vi "stopAllThreads.vi"(0 "HGF_ThreadPool":refnum<class "HGF_ThreadPool.lvclass">, 5 "error in (no error)":errorcluster) -> (14 "dup HGF_ThreadPool":refnum<class "HGF_ThreadPool.lvclass">, 19 "error out":errorcluster)   [LabVIEW 2014, in "HGF_BaseClasses.lvlib" / "HGF_ThreadPool.lvclass"]
doc: "Stop all threads of this ThreadPool."
uses:
  HGF_ThreadPool.lvclass
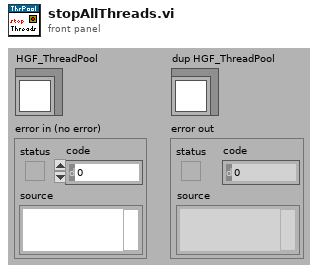
[diagram p1: front panel]
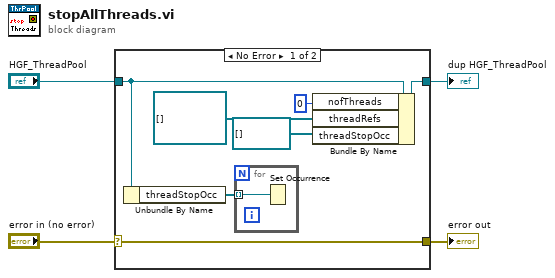
[diagram p0: block diagram]
diagram:
  n1 = case shown="No Error" "error in (no error)" {
    selector: "error in (no error)" -> [w11 w14]
    tunnel: [w11 w14] -> w3
    tunnel: [w8 w13] -> w1
    tunnel: "HGF_ThreadPool" -> [w9 w13]
    frame No Error {
      n2 = Unbundle By Name(w9) -> ("threadStopOcc"=w10:refnum<k4>[])
      n3 = for {
        tunnel: w10 -> [w12] mode=indexing
        n4 = Set Occurrence(w12) -> ()
      }
      n5 = Bundle By Name(cluster=w9, "nofThreads"=0, "threadRefs"=refnum<vi>[] [], "threadStopOcc"=refnum<k4>[] []) -> (w8:refnum<class "HGF_ThreadPool.lvclass">)
    }
    frame Error {
    }
  }
  "error out" <- w3
  "dup HGF_ThreadPool" <- w1
